vi "CheckTemperature.vi"(8 "error in (no error)":errorcluster, 11 "temperature in":i32) -> (0 "error out":errorcluster)   [LabVIEW 2013]
uses:
  Utilities/controls/ctlSeqFNs_Andor_temp.ctl
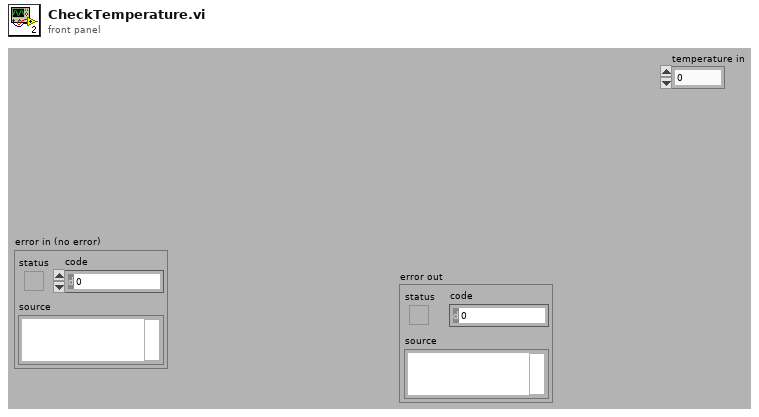
[diagram p1: front panel]
types:
  T1 = typedef "ctlSeqFNs_Andor_temp.ctl" = enum16{"Temperature  FALSE", "Temperature OK"}
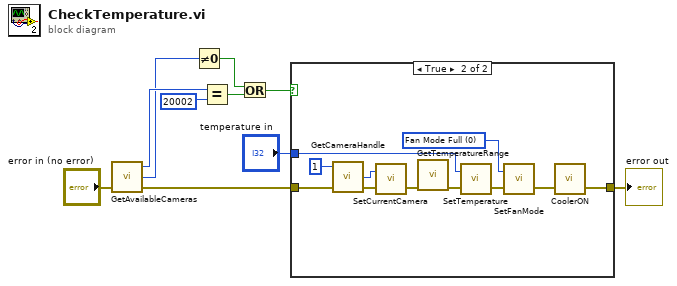
[diagram p0: block diagram]
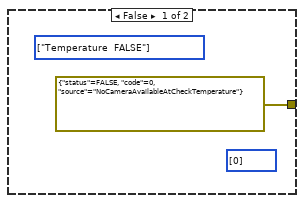
[diagram p2: hidden frame]
diagram:
  n1 = call "GetAvailableCameras.vi"("error in (no error)"="error in (no error)") -> ("error out"=w4:errorcluster, "totalCameras"=w3:i32, "DLL error code"=w10:u32)  [unwired: 2 in]
  n2 = Not Equal To 0?(x=w3) -> (x != 0?=w1:bool)
  n3 = Equal?(x=w10, y=u32 20002) -> (x = y?=w8:bool)
  n4 = Or(x=w1, y=w8) -> (x .or. y?=w6:bool)
  n5 = case shown="True" w6 {
    tunnel: [errorcluster {"status"=FALSE, "code"=0, "source"="NoCameraAvailableAtCheckTemperature"} ("error out") w22] -> w5
    tunnel: w4 -> [_ w21]
    tunnel: "temperature in" -> [_ w20]
    frame False {
      (unwired) i32[] [0]
      (unwired) T1[] [enum."Temperature  FALSE"] items=["Temperature  FALSE", "Temperature OK"]
    }
    frame True {
      w17 = u16 0 items=["Fan Mode Full", "Fan Mode Half", "Fan Mode Low"] ("Ring")
      n6 = call "GetCameraHandle.vi"("error in (no error)"=w21, "cameraIndex"=1) -> ("error out"=w16:errorcluster, "cameraHandle"=w15:i32)  [unwired: 1 in, 1 out]
      n7 = call "SetCurrentCamera.vi"("error in (no error)"=w16, "cameraHandle"=w15) -> ("error out"=w14:errorcluster)  [unwired: 1 out]
      n8 = call "GetTemperatureRange.vi"("error in (no error)"=w14) -> ("error out"=w19:errorcluster)  [unwired: 3 in, 3 out]
      n9 = call "SetTemperature.vi"("error in (no error)"=w19, "temperature"=w20) -> ("error out"=w18:errorcluster)  [unwired: 1 out]
      n10 = call "SetFanMode.vi"("error in (no error)"=w18, "mode"=w17) -> ("error out"=w12:errorcluster)  [unwired: 1 out]
      n11 = call "CoolerON.vi"("error in (no error)"=w12) -> ("error out"=w22:errorcluster)  [unwired: 1 in, 1 out]
    }
  }
  "error out" <- w5
